vi "_assert_name reuse2.vi"(7 "Name":string, 8 "error in (no error)":errorcluster) -> (0 "error out":errorcluster)   [LabVIEW 2020]
uses:
  classes/Assert/Assert.lvclass
  classes/Test/Test.lvclass
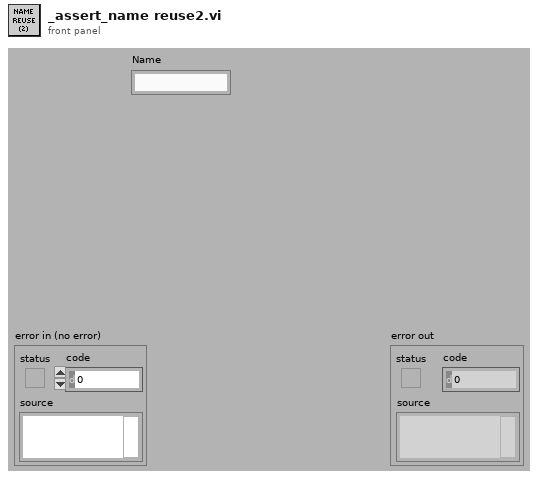
[diagram p1: front panel]
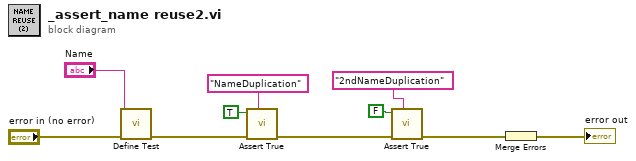
[diagram p0: block diagram]
diagram:
  n1 = call "Define Test.vi"("error in (no error)"="error in (no error)", "Label (VI Title)"="Name") -> ("error out"=w8:errorcluster)  [unwired: 8 in, 1 out]
  n2 = call "Assert True.vi"("Label"="NameDuplication", "error in (no error)"=w8, "True?"=TRUE) -> ("error out"=w3:errorcluster)  [unwired: 7 in, 1 out]
  n3 = call "Assert True.vi"("Label"="2ndNameDuplication", "error in (no error)"=w3, "True?"=FALSE) -> ("error out"=w2:errorcluster)  [unwired: 7 in, 1 out]
  n4 = Merge Errors(w2) -> (→"error out":errorcluster)
